vi "VCmodule.vi"(0 "input":tag="1/ai0, 1/ai4", 1 "output":tag="1/ao0", 2 "signal":dbl[](array[numeric]), 3 "piezo constant":dbl=1505.255 format="%#_13g", 4 "liczba probek":dbl=10000.0 min=100.0 max=1000000.0 step=10000.0, 5 "czas trwania [s]":dbl) -> (6 "PIEZO":dbl[](graph), 7 "psd":dbl[](graph), 8 "S/s":dbl)   [LabVIEW 2013]
uses:
  <vilib>/DAQmx/write.llb/DAQmx Write (Analog 1D DBL 1Chan NSamp).vi
  <vilib>/DAQmx/read.llb/DAQmx Read (Analog 2D DBL NChan NSamp).vi
  <vilib>/DAQmx/create/channels.llb/DAQmx Create Channel (AO-Voltage-Basic).vi
  <vilib>/DAQmx/configure/timing.llb/DAQmx Timing (Sample Clock).vi
  <vilib>/DAQmx/create/channels.llb/DAQmx Create Channel (AI-Voltage-Basic).vi
  <vilib>/DAQmx/configure/trigger.llb/DAQmx Start Trigger (Digital Edge).vi
  <vilib>/DAQmx/miscellaneous.llb/DAQmx Fill In Error Info.vi
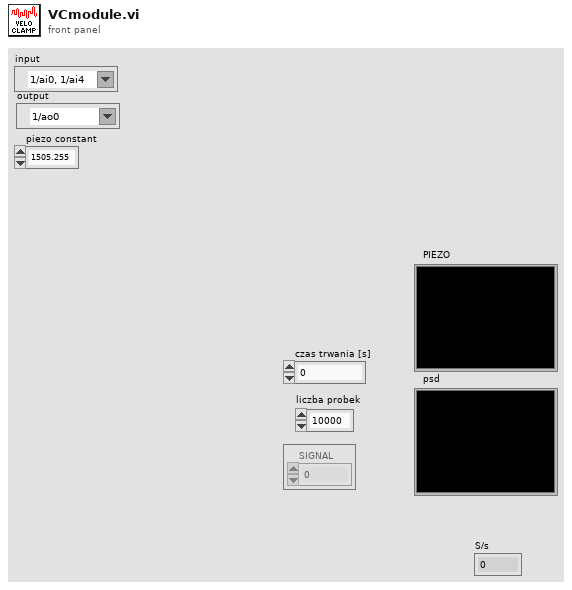
[diagram p1: front panel]
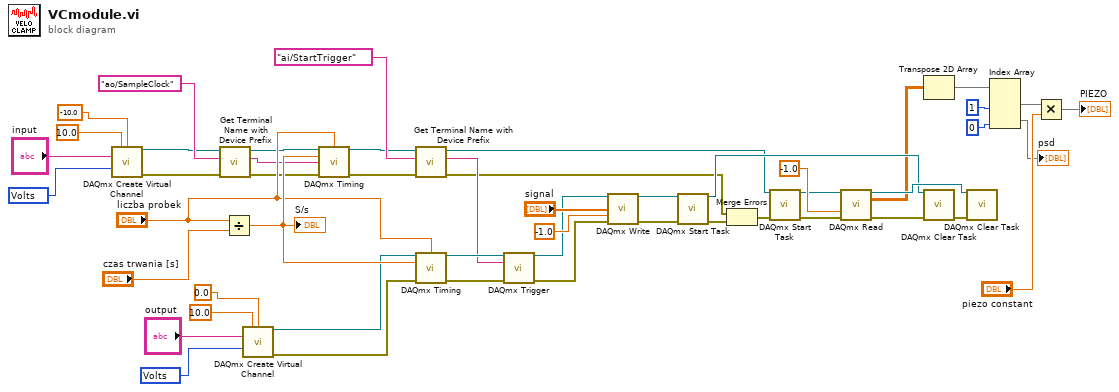
[diagram p0: block diagram]
diagram:
  w41 = 10348 items=["Volts"=10348, "From Custom Scale"=10065] ("units")
  w43 = 10348 items=["Volts"=10348, "From Custom Scale"=10065] ("units")
  n1 = call-poly <vilib>:"DAQmx Create Virtual Channel.vi"("maximum value"=10.0, "minimum value"=-10.0, "physical channels"="input", "units"=w41) -> ("task out"=w5:refnum<k21>, "error out"=w4:errorcluster)  [unwired: 10 in]
  n2 = call "Get Terminal Name with Device Prefix.vi"("error in (no error)"=w4, "Local Terminal Name"="ao/SampleClock", "task/channels in"=w5) -> ("error out"=w7:errorcluster, "Terminal Name with Device Prefix"=w1:tag, "task out"=w8:refnum<k21>)  [unwired: 6 in]
  n3 = Divide(x="liczba probek", y="czas trwania [s]") -> (x/y=w34:dbl)
  "S/s" <- w34
  n4 = call-poly <vilib>:"DAQmx Create Virtual Channel.vi"("maximum value"=10.0, "minimum value"=0.0, "physical channels"="output", "units"=w43) -> ("task out"=w3:refnum<k21>, "error out"=w2:errorcluster)  [unwired: 10 in]
  n5 = call-poly <vilib>:"DAQmx Timing.vi"("task/channels in"=w8, "samples per channel"="liczba probek", "rate"=w34, "source"=w1, "error in"=w7) -> ("task out"=w19:refnum<k21>, "error out"=w18:errorcluster)  [unwired: 9 in]
  n6 = call "Get Terminal Name with Device Prefix.vi"("error in (no error)"=w18, "Local Terminal Name"=tag "ai/StartTrigger" ("source"), "task/channels in"=w19) -> ("error out"=w15:errorcluster, "Terminal Name with Device Prefix"=w22:tag, "task out"=w17:refnum<k21>)  [unwired: 6 in]
  n7 = call-poly <vilib>:"DAQmx Timing.vi"("task/channels in"=w3, "samples per channel"="liczba probek", "rate"=w34, "error in"=w2) -> ("task out"=w25:refnum<k21>, "error out"=w24:errorcluster)  [unwired: 10 in]
  n8 = call-poly <vilib>:"DAQmx Trigger.vi"("task/channels in"=w25, "source"=w22, "error in"=w24) -> ("task out"=w20:refnum<k21>, "error out"=w21:errorcluster)  [unwired: 11 in]
  n9 = call-poly <vilib>:"DAQmx Write.vi"("task/channels in"=w20, "data"="signal", "timeout"=-1.0, "error in"=w21) -> ("task out"=w49:refnum<k21>, "error out"=w16:errorcluster)  [unwired: 9 in, 1 out]
  n10 = call <vilib>:"DAQmx Start Task.vi"("task/channels in"=w49, "error in"=w16) -> ("task out"=w36:refnum<k21>, "error out"=w14:errorcluster)  [unwired: 12 in]
  n11 = Merge Errors(w15, w14) -> (w13:errorcluster)
  n12 = call <vilib>:"DAQmx Start Task.vi"("task/channels in"=w17, "error in"=w13) -> ("task out"=w12:refnum<k21>, "error out"=w11:errorcluster)  [unwired: 12 in]
  n13 = call-poly <vilib>:"DAQmx Read.vi"("task/channels in"=w12, "timeout"=-1.0, "error in"=w11) -> ("task out"=w37:refnum<k21>, "data"=w33:dbl[][], "error out"=w38:errorcluster)  [unwired: 10 in]
  n14 = Transpose 2D Array(2D array=w33) -> (transposed array=w31:dbl[][])
  n15 = call <vilib>:"DAQmx Clear Task.vi"("task in"=w36, "error in"=w38) -> ("error out"=w10:errorcluster)  [unwired: 13 in]
  n16 = call <vilib>:"DAQmx Clear Task.vi"("task in"=w37, "error in"=w10) -> ()  [unwired: 13 in, 1 out]
  n17 = Index Array(array=w31, index (col) #1=1 ("index"), index (col) #2=0 ("index")) -> (element #1=w29:dbl[], element #2=→"psd":dbl[])  [unwired: 2 in]
  n18 = Multiply(x=w29, y="piezo constant") -> (x*y=→"PIEZO":dbl[])
